vi "bubbleSort.vi"() -> ()   [LabVIEW 2014]
doc: "Bubble Sort"
panel:
  out "Bubble Sort Waveform bar graph":dbl[](graph)
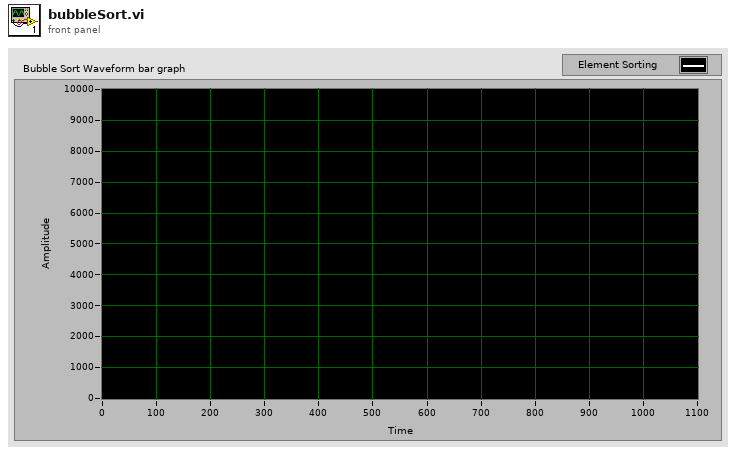
[diagram p1: front panel]
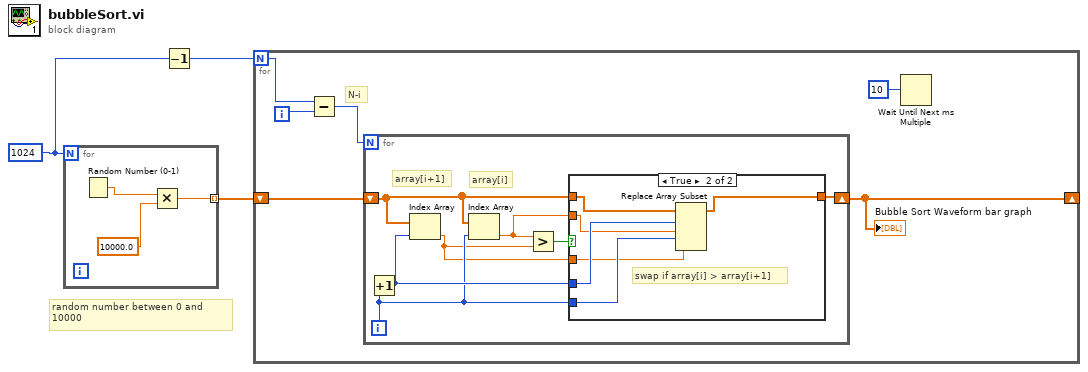
[diagram p0: block diagram]
diagram:
  w1 = 1024
  # "random number between 0 and\n10000"
  n1 = for {
    N: w1 -> [_]
    tunnel: [w4] -> w3 mode=indexing
    n2 = Random Number (0-1)() -> (number: 0 to 1=w6:dbl)
    n3 = Multiply(x=w6, y=10000.0) -> (x*y=w4:dbl)
  }
  n4 = Decrement(x=w1) -> (x-1=w2:i32)
  n5 = for {
    N: w2 -> [w12]
    shift-right: [w8] -> _
    shift-left: w3 -> [w9]
    i -> [w11]
    # "N-i"
    n6 = Subtract(x=w12, y=w11) -> (x-y=w10:i32)
    n7 = for {
      N: w10 -> [_]
      shift-right: [w17] -> w8
      shift-left: w9 -> [w19]
      i -> [w15]
      # "array[i]"
      # "array[i+1]"
      n8 = Increment(x=w15) -> (x+1=w16:i32)
      n9 = Index Array(array=w19, index=w16) -> (element=w13:dbl)
      n10 = Index Array(array=w19, index=w15) -> (element=w14:dbl)
      n11 = Greater?(x=w14, y=w13) -> (0:w18:bool)
      n12 = case shown="True" w18 {
        tunnel: w19 -> [w20 w22]
        tunnel: [w20 w21] -> w17
        tunnel: w15 -> [_ w25]
        tunnel: w16 -> [_ w26]
        tunnel: w14 -> [_ w24]
        tunnel: w13 -> [_ w23]
        frame False {
        }
        frame True {
          # "swap if array[i] > array[i+1]"
          n13 = Replace Array Subset(array=w22, new element #1=w24, index #1=w26, new element #2=w23, index #2=w25) -> (w21:dbl[])
        }
      }
    }
    "Bubble Sort Waveform bar graph" <- w8
    n14 = Wait Until Next ms Multiple(millisecond multiple=10) -> ()  [unwired: 1 out]
  }
